vi "Parse Sensors Data.vi"(8 "error in":errorcluster, 11 "Data":string) -> (0 "error out":errorcluster, 3 "Sensors Data":T1={"Temperature (°C)"=nan, "Barometric Pressure (mbar)"=nan, "Humidity (%)"=nan, "Temperature Cooler (K)"=nan})   [LabVIEW 2019, in "ACSVcontrol-driver.lvlib"]
doc: "Parse data recieved from PJVS with sensor data."
uses:
  ACSVcontrol-driver.lvlib
  Public/Type Definitions/Sensors Data.ctl
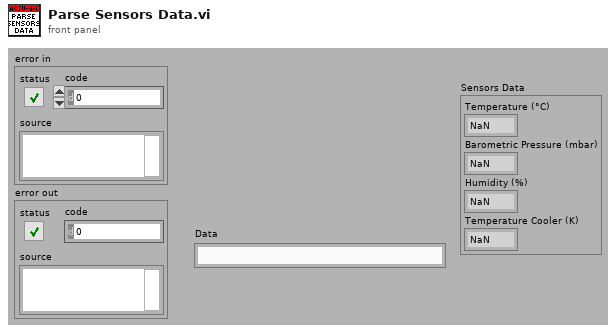
[diagram p1: front panel]
types:
  T1 = typedef "ACSVcontrol-driver.lvlib/Sensors Data.ctl" = cluster{"Temperature (°C)":dbl, "Barometric Pressure (mbar)":dbl, "Humidity (%)":dbl, "Temperature Cooler (K)":dbl}
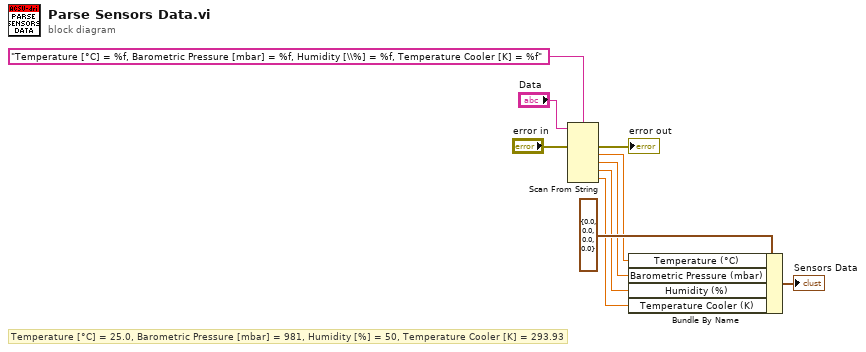
[diagram p0: block diagram]
diagram:
  # "Temperature [°C] = 25.0, Barometric Pressure [mbar] = 981, Humidity [%] = 50, Temperature Cooler [K] = 293.93"
  n1 = Scan From String(format string="Temperature [°C] = %f, Barometric Pressure [mbar] = %f, Humidity [\\%] = %f, Temperature Cooler [K] = %f", input string="Data", error in="error in") -> (error out=→"error out":errorcluster, output 1=w8:dbl, output 2=w7:dbl, output 3=w6:dbl, output 4=w5:dbl)  [unwired: 5 in, 2 out]
  n2 = Bundle By Name(cluster=T1 {"Temperature (°C)"=0.0, "Barometric Pressure (mbar)"=0.0, "Humidity (%)"=0.0, "Temperature Cooler (K)"=0.0} ("Snsors Data"), "Temperature (°C)"=w8, "Barometric Pressure (mbar)"=w7, "Humidity (%)"=w6, "Temperature Cooler (K)"=w5) -> (→"Sensors Data":T1)
